vi "Create HDU.vi"(8 "error in (no error)":errorcluster, 11 "Save Image in":refnum<class "Save Image.lvclass">) -> (0 "error out":errorcluster, 3 "Save Image out":refnum<class "Save Image.lvclass">)   [LabVIEW 2018, in "Save Image.lvclass"]
uses:
  Save Image.lvclass
  Simulated_Header/Simulated_Header.lvclass
  Interface/Interface.lvclass
  <userlib>/gfitsio/cfitsio-bitpix.ctl
  <userlib>/gfitsio/gfitsio.lvlib
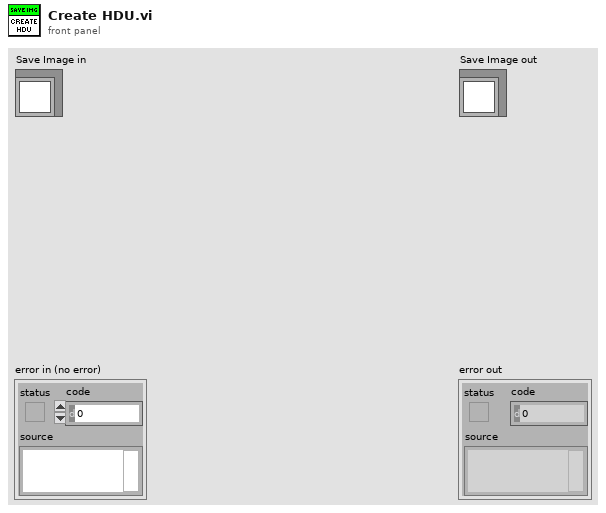
[diagram p1: front panel]
types:
  T1 = enum16{"open", "open or create", "create", "create or replace"}
  T2 = typedef "gfitsio.lvlib/cfitsio-bitpix.ctl" = i32
  T3 = cluster{"PREAMP":u16, "READOUT_RATE":u16, "EM_GAIN":u16, "VBIN":u16, "INITIAL_LINE":u16, "INITIAL_COLUMN":u16, "FINAL_LINE":u16, "FINAL_COLUMN":u16, "TRIGGER_MODE":u16, "HBIN":u16, "SHUTTER_TTL":u16, "SHUTTER_MODE":u16, "SHUTTER_OPENING_TIME":u16, "SHUTTER_CLOSING_TIME":u16, "VERTICAL_SHIFT_SPEED":u16, "READ_MODE":u16, "FRAME_TRANSFER":bool, "VERTICAL_CLOCK_VOLTAGE":u16, "ACQUISITION_MODE":u16, "AD_CHANNEL":u16, "EM_MODE":u16}
  T4 = typedef "gfitsio.lvlib/gfitsio-refnum.ctl" = refnum<k1>
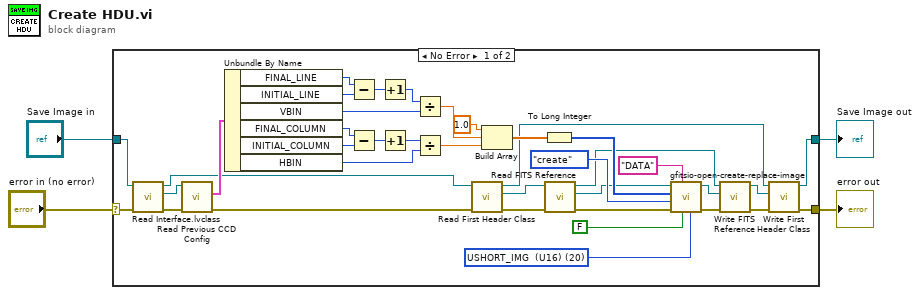
[diagram p0: block diagram]
diagram:
  n1 = case shown="No Error" "error in (no error)" {
    selector: "error in (no error)" -> [w11 w44]
    tunnel: [w20 w44] -> w3
    tunnel: [w24 w43] -> w1
    tunnel: "Save Image in" -> [w15 w43]
    frame No Error {
      w40 = T2 20 items=["<invalid type>"=0, "BYTE_IMG  (U8)"=8, "SHORT_IMG  (I16)"=16, "USHORT_IMG  (U16)"=20, "LONG_IMG  (I32)"=32, "ULONG_IMG  (U32)"=40, "FLOAT_IMG  (SGL)"=-32, "DOUBLE_IMG  (DBL)"=-64] ("image data type")
      n2 = call "Read Interface.lvclass.vi"("error in (no error)"=w11, "Save Image in"=w15) -> ("error out"=w17:errorcluster, "Interface.lvclass"=w18:refnum<class "Interface.lvclass">, "Save Image out"=w9:refnum<class "Save Image.lvclass">)  [unwired: 7 in]
      n3 = call "Read Previous CCD Config.vi"("error in (no error)"=w17, "Interface in"=w18) -> ("error out"=w10:errorcluster, "CCD Config"=w19:T3)  [unwired: 7 in, 1 out]
      n4 = Unbundle By Name(w19) -> ("FINAL_LINE"=w30:u16, "INITIAL_LINE"=w29:u16, "VBIN"=w28:u16, "FINAL_COLUMN"=w27:u16, "INITIAL_COLUMN"=w26:u16, "HBIN"=w25:u16)
      n5 = Subtract(x=w30, y=w29) -> (x-y=w37:u16)
      n6 = Subtract(x=w27, y=w26) -> (x-y=w38:u16)
      n7 = Increment(x=w37) -> (x+1=w36:u16)
      n8 = Increment(x=w38) -> (x+1=w35:u16)
      n9 = Divide(x=w36, y=w28) -> (x/y=w34:dbl)
      n10 = Divide(x=w35, y=w25) -> (x/y=w33:dbl)
      n11 = call "Read First Header Class.vi"("error in (no error)"=w10, "Save Image in"=w9) -> ("error out"=w7:errorcluster, "Simulated_Header.lvclass"=w6:refnum<class "Simulated_Header.lvclass">, "Save Image out"=w8:refnum<class "Save Image.lvclass">)  [unwired: 7 in]
      n12 = Build Array(1.0 ("element"), w34, w33) -> (w32:dbl[])
      n13 = To Long Integer(number=w32) -> (32bit integer=w31:i32[])
      n14 = call "Read FITS Reference.vi"("error in (no error)"=w7, "Simulated_Header in"=w6) -> ("error out"=w13:errorcluster, "gfits refnum"=w14:T4, "Simulated_Header out"=w12:refnum<class "Simulated_Header.lvclass">)  [unwired: 7 in]
      n15 = call <userlib>:"gfitsio-open-create-replace-image.vi"("image data type"=w40, "advisory dialog? (display:T)"=FALSE, "hdu name (dialog if empty)"="DATA" ("prompt"), "error in (no error)"=w13, "function (create or replace)"=T1."create" ("function (open or create)"), "naxes"=w31, "gfits refnum"=w14) -> ("error out"=w16:errorcluster, "dup gfits refnum"=w23:T4)  [unwired: 2 in, 1 out]
      n16 = call "Write FITS Reference.vi"("error in (no error)"=w16, "gfits refnum"=w23, "Simulated_Header in"=w12) -> ("error out"=w21:errorcluster, "Simulated_Header out"=w22:refnum<class "Simulated_Header.lvclass">)  [unwired: 7 in]
      n17 = call "Write First Header Class.vi"("error in (no error)"=w21, "Simulated_Header.lvclass"=w22, "Save Image in"=w8) -> ("error out"=w20:errorcluster, "Save Image out"=w24:refnum<class "Save Image.lvclass">)  [unwired: 7 in]
    }
    frame Error {
    }
  }
  "error out" <- w3
  "Save Image out" <- w1
